vi "DAQNavi Read (Analog DBL 1Chan 1Samp).vi"(8 "error in (no error)":errorcluster, 10 "timeout":dbl=10.0, 11 "task in":i32) -> (0 "error out":errorcluster, 2 "data":dbl, 3 "task out":i32)   [LabVIEW 2020]
uses:
  DAQNavi_LV.dll
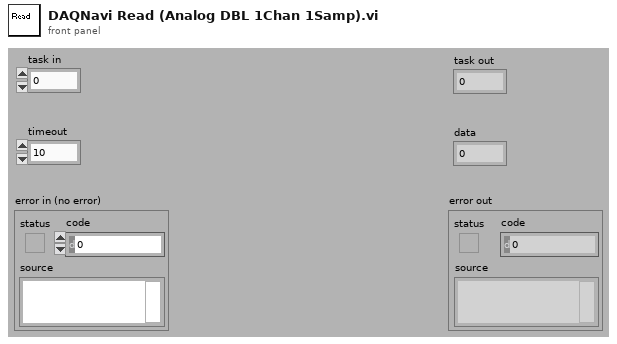
[diagram p1: front panel]
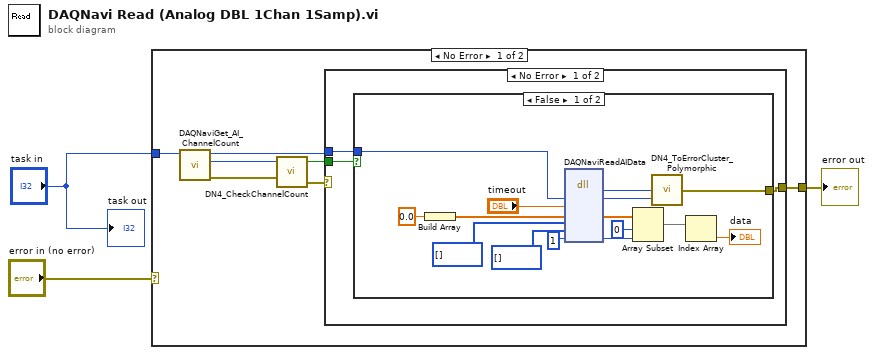
[diagram p0: block diagram]
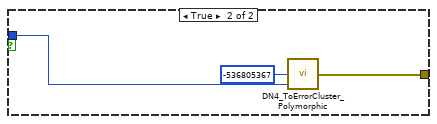
[diagram p2: hidden frame]
diagram:
  n1 = case shown="No Error" "error in (no error)" {
    selector: "error in (no error)" -> [_ w33]
    tunnel: "task in" -> [w10 _]
    tunnel: [w9 w33] -> w2
    frame No Error {
      n2 = call "DAQNaviGet_AI_ChannelCount.vi"("task in"=w10) -> ("error out"=w7:errorcluster, "channel count"=w8:i32, "task out"=w4:i32)  [unwired: 1 in, 7 out]
      n3 = call "DN4_CheckChannelCount.vi"("error out"=w7, "channel count"=w8) -> ("error IO"=w5:errorcluster, "greater than 1?"=w6:bool)  [unwired: 2 out]
      n4 = case shown="No Error" w5 {
        selector: w5 -> [_ w32]
        tunnel: w6 -> [w13 _]
        tunnel: [w12 w32] -> w9
        tunnel: w4 -> [w11 _]
        frame No Error {
          n5 = case shown="False" w13 {
            tunnel: [w20 w30] -> w12
            tunnel: w11 -> [w19 w29]
            frame False {
              n6 = Build Array(0.0 ("element")) -> (w23:dbl[])
              n7 = dll-call lib="DAQNavi_LV.dll" fn="DAQNaviReadAIData"("taskID"=w19, "timeout"="timeout", "scaledData"=w23, "rawData16"=u16[] [], "rawData32"=u32[] [], "samples"=u32 1) -> ("return type"=w21:i32, "taskID"=w14:i32, "scaledData"=w18:dbl[], "samples"=w16:u32)  [unwired: 4 in, 4 out]
              n8 = Array Subset(array=w18, index=0, length=w16) -> (w15:dbl[])
              n9 = call "DN4_ToErrorCluster_Polymorphic.vi"("task id"=w14, "error code"=w21) -> ("error out"=w20:errorcluster)  [unwired: 3 out]
              n10 = Index Array(array=w15) -> (element=→"data":dbl)  [unwired: 1 in]
            }
            frame True {
              n11 = call "DN4_ToErrorCluster_Polymorphic.vi"("task id"=w29, "error code"=-536805367 ("error code (0)")) -> ("error out"=w30:errorcluster)  [unwired: 3 out]
            }
          }
        }
        frame Error {
        }
      }
    }
    frame Error {
    }
  }
  "error out" <- w2
  "task out" <- "task in"
